vi "Parse Token.vi"(7 "Loader":refnum<class "Abstract.lvclass">, 8 "Error In":errorcluster, 10 "Token":refnum<class "Abstract.lvclass">, 11 "Stack In":refnum<queue>) -> (0 "Error Out":errorcluster, 3 "Stack Out":refnum<queue>)   [LabVIEW 2018, in "Toolkit.lvlib"]
uses:
  Toolkit.lvlib
  Nodes/NonTerminal/NonTerminal.lvclass
  D:/Users/cfield/Code/Field R&D Services/Mustache/LabVIEW/trunk/src/Toolkit/Low-Level/Nodes/Abstract/Abstract.lvclass
  Tokens/Abstract/Abstract.lvclass
  Loaders/Abstract/Abstract.lvclass
  Tokens/Comment/Comment.lvclass
  Tokens/SetDelimiter/SetDelimiter.lvclass
  Tokens/SetDelimiter/SetDelimiter.lvclass/SetDelimiter.ctl
  Tokens/Text/Text.lvclass
  Nodes/Section/Section.lvclass
  D:/Users/cfield/Code/Field R&D Services/Mustache/LabVIEW/trunk/src/Toolkit/Low-Level/Nodes/NonTerminal/NonTerminal.lvclass
  Nodes/Comment/Comment.lvclass
  Nodes/Tag/Tag.lvclass
  Nodes/Partial/Partial.lvclass
  Nodes/Delimiter/Delimiter.lvclass
  Nodes/Text/Text.lvclass
  Lex String.vi
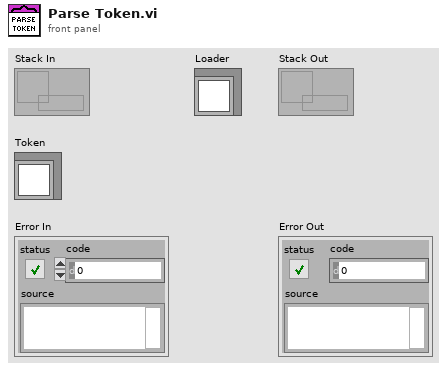
[diagram p1: front panel]
types:
  T1 = typedef "Toolkit.lvlib/Delimiters.ctl" = cluster{"Close":string, "Open":string}
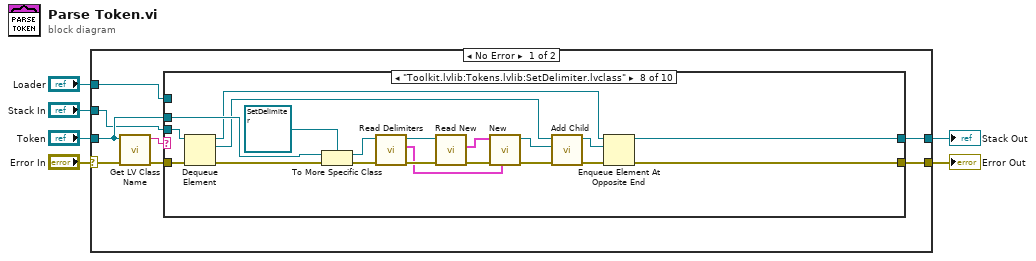
[diagram p0: block diagram]
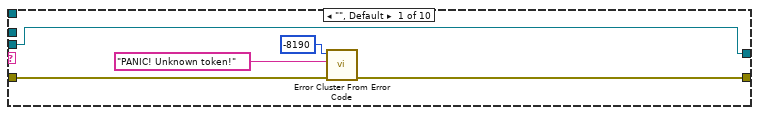
[diagram p2: hidden frame]
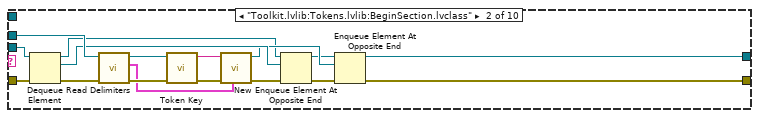
[diagram p3: hidden frame]
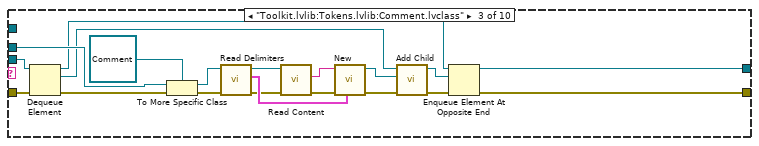
[diagram p4: hidden frame]
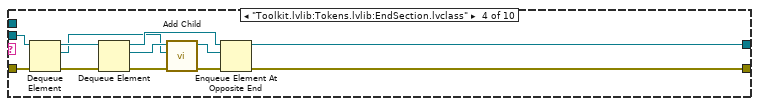
[diagram p5: hidden frame]
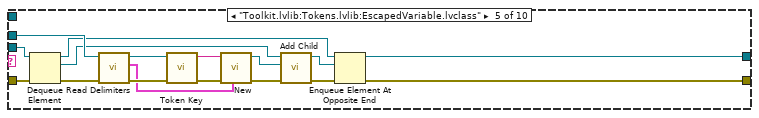
[diagram p6: hidden frame]
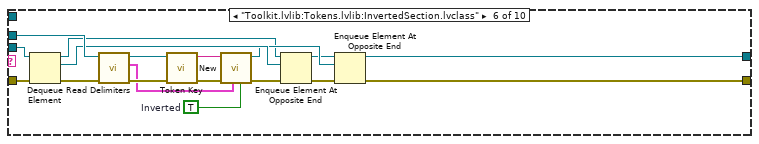
[diagram p7: hidden frame]
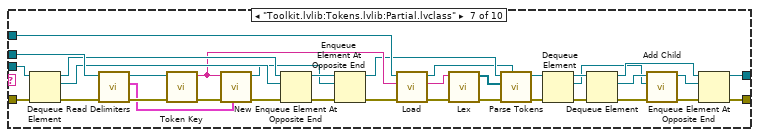
[diagram p8: hidden frame]
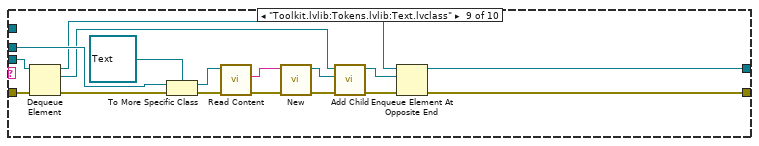
[diagram p9: hidden frame]
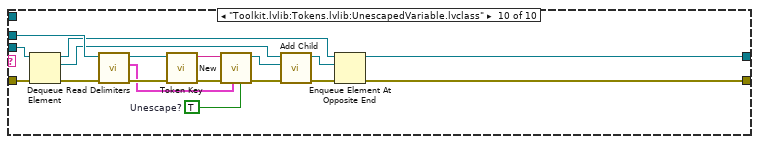
[diagram p10: hidden frame]
diagram:
  n1 = case shown="No Error" "Error In" {
    selector: "Error In" -> [w9 w194]
    tunnel: [w14 w195] -> w6
    tunnel: "Token" -> [w13 _]
    tunnel: [w12 w194] -> w4
    tunnel: "Stack In" -> [w8 w195]
    tunnel: "Loader" -> [w7 _]
    frame No Error {
      n2 = call <vilib>:"Get LV Class Name.vi"("error in (no error)"=w9, "object"=w13) -> ("error out"=w11:errorcluster, "class name"=w10:string)  [unwired: 8 in]
      n3 = case shown="\"Toolkit.lvlib:Tokens.lvlib:SetDelimiter.lvclass\"" w10 {
        tunnel: w11 -> [w19 w33 w56 w68 w85 w100 w136 w158 w175 w191]
        tunnel: [w17 w31 w46 w58 w75 w98 w115 w149 w164 w182] -> w12
        tunnel: w13 -> [_ w36 w55 _ w84 w103 w138 w157 w173 w190]
        tunnel: w8 -> [w15 w34 w52 w67 w81 w101 w137 w155 w170 w188]
        tunnel: [w15 w30 w49 w60 w78 w97 w116 w152 w167 w185] -> w14
        tunnel: w7 -> [_ _ _ _ _ _ w114 _ _ _]
        frame "", Default {
          n4 = call <vilib>:"Error Cluster From Error Code.vi"("error in (no error)"=w19, "error message (\"\")"="PANIC! Unknown token!" ("error message (\"\")"), "error code (0)"=-8190) -> ("error out"=w17:errorcluster)  [unwired: 6 in]
        }
        frame "Toolkit.lvlib:Tokens.lvlib:BeginSection.lvclass" {
          n5 = Dequeue Element(queue=w34, error in (no error)=w33) -> (queue out=w28:refnum<queue>, element=w32:refnum<class "NonTerminal.lvclass">, error out=w22:errorcluster)  [unwired: 1 in, 1 out]
          n6 = call-dynamic "Read Delimiters.vi"("Error In"=w22, "Token In"=w36) -> ("Error Out"=w21:errorcluster, "Delimiters"=w20:T1, "Token Out"=w23:refnum<class "Abstract.lvclass">)  [unwired: 7 in]
          n7 = call "Token Key.vi"("Error In"=w21, "Token"=w23) -> ("Error Out"=w25:errorcluster, "Key"=w35:string)  [unwired: 8 in]
          n8 = call "New.vi"("Delimiters"=w20, "Error In"=w25, "Key"=w35) -> ("Error Out"=w24:errorcluster, "Section"=w29:refnum<class "Section.lvclass">)  [unwired: 7 in]
          n9 = Enqueue Element At Opposite End(queue=w28, element=w32, error in (no error)=w24) -> (queue out=w27:refnum<queue>, error out=w26:errorcluster)  [unwired: 1 in, 1 out]
          n10 = Enqueue Element At Opposite End(queue=w27, element=w29, error in (no error)=w26) -> (queue out=w30:refnum<queue>, error out=w31:errorcluster)  [unwired: 1 in, 1 out]
        }
        frame "Toolkit.lvlib:Tokens.lvlib:Comment.lvclass" {
          n11 = Dequeue Element(queue=w52, error in (no error)=w56) -> (queue out=w50:refnum<queue>, element=w51:refnum<class "NonTerminal.lvclass">, error out=w53:errorcluster)  [unwired: 1 in, 1 out]
          n12 = To More Specific Class(target class=refnum<class "Comment.lvclass"> refnum ("Toolkit.lvlib:Tokens.lvlib:Comment.lvclass"), reference=w55, error in=w53) -> (specific class reference=w41:refnum<class "Comment.lvclass">, error out=w37:errorcluster)
          n13 = call-dynamic "Read Delimiters.vi"("Error In"=w37, "Token In"=w41) -> ("Error Out"=w38:errorcluster, "Delimiters"=w42:T1, "Token Out"=w40:refnum<class "Comment.lvclass">)  [unwired: 7 in]
          n14 = call-dynamic "Read Content.vi"("Error In"=w38, "Contentable In"=w40) -> ("Error Out"=w39:errorcluster, "Content"=w43:string)  [unwired: 7 in, 1 out]
          n15 = call "New.vi"("Delimiters"=w42, "Error In"=w39, "Content"=w43) -> ("Error Out"=w44:errorcluster, "Comment"=w54:refnum<class "Comment.lvclass">)  [unwired: 7 in]
          n16 = call-dynamic "Add Child.vi"("Error In"=w44, "Child"=w54, "Non-Terminal In"=w51) -> ("Error Out"=w47:errorcluster, "Non-Terminal Out"=w48:refnum<class "NonTerminal.lvclass">)  [unwired: 7 in]
          n17 = Enqueue Element At Opposite End(queue=w50, element=w48, error in (no error)=w47) -> (queue out=w49:refnum<queue>, error out=w46:errorcluster)  [unwired: 1 in, 1 out]
        }
        frame "Toolkit.lvlib:Tokens.lvlib:EndSection.lvclass" {
          n18 = Dequeue Element(queue=w67, error in (no error)=w68) -> (queue out=w66:refnum<queue>, element=w62:refnum<class "NonTerminal.lvclass">, error out=w64:errorcluster)  [unwired: 1 in, 1 out]
          n19 = Dequeue Element(queue=w66, error in (no error)=w64) -> (queue out=w65:refnum<queue>, element=w63:refnum<class "NonTerminal.lvclass">, error out=w61:errorcluster)  [unwired: 1 in, 1 out]
          n20 = call-dynamic "Add Child.vi"("Error In"=w61, "Child"=w62, "Non-Terminal In"=w63) -> ("Error Out"=w59:errorcluster, "Non-Terminal Out"=w57:refnum<class "NonTerminal.lvclass">)  [unwired: 7 in]
          n21 = Enqueue Element At Opposite End(queue=w65, element=w57, error in (no error)=w59) -> (queue out=w60:refnum<queue>, error out=w58:errorcluster)  [unwired: 1 in, 1 out]
        }
        frame "Toolkit.lvlib:Tokens.lvlib:EscapedVariable.lvclass" {
          n22 = Dequeue Element(queue=w81, error in (no error)=w85) -> (queue out=w79:refnum<queue>, element=w80:refnum<class "NonTerminal.lvclass">, error out=w71:errorcluster)  [unwired: 1 in, 1 out]
          n23 = call-dynamic "Read Delimiters.vi"("Error In"=w71, "Token In"=w84) -> ("Error Out"=w70:errorcluster, "Delimiters"=w69:T1, "Token Out"=w72:refnum<class "Abstract.lvclass">)  [unwired: 7 in]
          n24 = call "Token Key.vi"("Error In"=w70, "Token"=w72) -> ("Error Out"=w74:errorcluster, "Key"=w82:string)  [unwired: 8 in]
          n25 = call "New.vi"("Delimiters"=w69, "Error In"=w74, "Key"=w82) -> ("Error Out"=w73:errorcluster, "Tag"=w83:refnum<class "Tag.lvclass">)  [unwired: 7 in]
          n26 = call-dynamic "Add Child.vi"("Error In"=w73, "Child"=w83, "Non-Terminal In"=w80) -> ("Error Out"=w76:errorcluster, "Non-Terminal Out"=w77:refnum<class "NonTerminal.lvclass">)  [unwired: 7 in]
          n27 = Enqueue Element At Opposite End(queue=w79, element=w77, error in (no error)=w76) -> (queue out=w78:refnum<queue>, error out=w75:errorcluster)  [unwired: 1 in, 1 out]
        }
        frame "Toolkit.lvlib:Tokens.lvlib:InvertedSection.lvclass" {
          w92 = TRUE  # Inverted
          n28 = Dequeue Element(queue=w101, error in (no error)=w100) -> (queue out=w95:refnum<queue>, element=w99:refnum<class "NonTerminal.lvclass">, error out=w88:errorcluster)  [unwired: 1 in, 1 out]
          n29 = call-dynamic "Read Delimiters.vi"("Error In"=w88, "Token In"=w103) -> ("Error Out"=w87:errorcluster, "Delimiters"=w86:T1, "Token Out"=w89:refnum<class "Abstract.lvclass">)  [unwired: 7 in]
          n30 = call "Token Key.vi"("Error In"=w87, "Token"=w89) -> ("Error Out"=w91:errorcluster, "Key"=w102:string)  [unwired: 8 in]
          n31 = call "New.vi"("Inverted"=w92, "Delimiters"=w86, "Error In"=w91, "Key"=w102) -> ("Error Out"=w90:errorcluster, "Section"=w96:refnum<class "Section.lvclass">)  [unwired: 6 in]
          n32 = Enqueue Element At Opposite End(queue=w95, element=w99, error in (no error)=w90) -> (queue out=w94:refnum<queue>, error out=w93:errorcluster)  [unwired: 1 in, 1 out]
          n33 = Enqueue Element At Opposite End(queue=w94, element=w96, error in (no error)=w93) -> (queue out=w97:refnum<queue>, error out=w98:errorcluster)  [unwired: 1 in, 1 out]
        }
        frame "Toolkit.lvlib:Tokens.lvlib:Partial.lvclass" {
          n34 = Dequeue Element(queue=w137, error in (no error)=w136) -> (queue out=w134:refnum<queue>, element=w135:refnum<class "NonTerminal.lvclass">, error out=w130:errorcluster)  [unwired: 1 in, 1 out]
          n35 = call-dynamic "Read Delimiters.vi"("Error In"=w130, "Token In"=w138) -> ("Error Out"=w129:errorcluster, "Delimiters"=w125:T1, "Token Out"=w131:refnum<class "Abstract.lvclass">)  [unwired: 7 in]
          n36 = call "Token Key.vi"("Error In"=w129, "Token"=w131) -> ("Error Out"=w128:errorcluster, "Key"=w112:string)  [unwired: 8 in]
          n37 = call "New.vi"("Delimiters"=w125, "Error In"=w128, "Key"=w112) -> ("Error Out"=w127:errorcluster, "Partial"=w126:refnum<class "Partial.lvclass">)  [unwired: 7 in]
          n38 = Enqueue Element At Opposite End(queue=w134, element=w135, error in (no error)=w127) -> (queue out=w133:refnum<queue>, error out=w132:errorcluster)  [unwired: 1 in, 1 out]
          n39 = Enqueue Element At Opposite End(queue=w133, element=w126, error in (no error)=w132) -> (queue out=w107:refnum<queue>, error out=w113:errorcluster)  [unwired: 1 in, 1 out]
          n40 = call-dynamic "Load.vi"("Error In"=w113, "Key"=w112, "Loader In"=w114) -> ("Error Out"=w105:errorcluster, "Template"=w106:string, "Loader Out"=w104:refnum<class "Abstract.lvclass">)  [unwired: 6 in]
          n41 = call-poly "Lex.vi"("Error In"=w105, "Input"=w106) -> ("Error Out"=w111:errorcluster, "Tokens"=w110:refnum<class "Abstract.lvclass">[])  [unwired: 8 in]
          n42 = call "Parse Tokens.vi"("Loader"=w104, "Error In"=w111, "Tokens"=w110, "Stack In"=w107) -> ("Error Out"=w109:errorcluster, "Stack Out"=w108:refnum<queue>)  [unwired: 6 in]
          n43 = Dequeue Element(queue=w108, error in (no error)=w109) -> (queue out=w124:refnum<queue>, element=w120:refnum<class "NonTerminal.lvclass">, error out=w122:errorcluster)  [unwired: 1 in, 1 out]
          n44 = Dequeue Element(queue=w124, error in (no error)=w122) -> (queue out=w123:refnum<queue>, element=w121:refnum<class "NonTerminal.lvclass">, error out=w119:errorcluster)  [unwired: 1 in, 1 out]
          n45 = call-dynamic "Add Child.vi"("Error In"=w119, "Child"=w120, "Non-Terminal In"=w121) -> ("Error Out"=w118:errorcluster, "Non-Terminal Out"=w117:refnum<class "NonTerminal.lvclass">)  [unwired: 7 in]
          n46 = Enqueue Element At Opposite End(queue=w123, element=w117, error in (no error)=w118) -> (queue out=w116:refnum<queue>, error out=w115:errorcluster)  [unwired: 1 in, 1 out]
        }
        frame "Toolkit.lvlib:Tokens.lvlib:SetDelimiter.lvclass" {
          n47 = Dequeue Element(queue=w155, error in (no error)=w158) -> (queue out=w153:refnum<queue>, element=w154:refnum<class "NonTerminal.lvclass">, error out=w156:errorcluster)  [unwired: 1 in, 1 out]
          n48 = To More Specific Class(target class=refnum<class "SetDelimiter.lvclass"> refnum ("Toolkit.lvlib:Tokens.lvlib:SetDelimiter.lvclass"), reference=w157, error in=w156) -> (specific class reference=w148:refnum<class "SetDelimiter.lvclass">, error out=w147:errorcluster)
          n49 = call-dynamic "Read Delimiters.vi"("Error In"=w147, "Token In"=w148) -> ("Error Out"=w145:errorcluster, "Delimiters"=w139:T1, "Token Out"=w144:refnum<class "SetDelimiter.lvclass">)  [unwired: 7 in]
          n50 = call "Read New.vi"("Error In"=w145, "SetDelimiter In"=w144) -> ("Error Out"=w143:errorcluster, "New Value"=w140:cluster{"Close":string, "Open":string})  [unwired: 7 in, 1 out]
          n51 = call "New.vi"("Delimiters"=w139, "Error In"=w143, "New Delimiters"=w140) -> ("Error Out"=w142:errorcluster, "Delimiter"=w141:refnum<class "Delimiter.lvclass">)  [unwired: 7 in]
          n52 = call-dynamic "Add Child.vi"("Error In"=w142, "Child"=w141, "Non-Terminal In"=w154) -> ("Error Out"=w150:errorcluster, "Non-Terminal Out"=w151:refnum<class "NonTerminal.lvclass">)  [unwired: 7 in]
          n53 = Enqueue Element At Opposite End(queue=w153, element=w151, error in (no error)=w150) -> (queue out=w152:refnum<queue>, error out=w149:errorcluster)  [unwired: 1 in, 1 out]
        }
        frame "Toolkit.lvlib:Tokens.lvlib:Text.lvclass" {
          n54 = Dequeue Element(queue=w170, error in (no error)=w175) -> (queue out=w168:refnum<queue>, element=w169:refnum<class "NonTerminal.lvclass">, error out=w171:errorcluster)  [unwired: 1 in, 1 out]
          n55 = To More Specific Class(target class=refnum<class "Text.lvclass"> refnum ("Toolkit.lvlib:Tokens.lvlib:Text.lvclass"), reference=w173, error in=w171) -> (specific class reference=w162:refnum<class "Text.lvclass">, error out=w161:errorcluster)
          n56 = call-dynamic "Read Content.vi"("Error In"=w161, "Contentable In"=w162) -> ("Error Out"=w159:errorcluster, "Content"=w160:string)  [unwired: 7 in, 1 out]
          n57 = call "New.vi"("Error In"=w159, "Content"=w160) -> ("Error Out"=w163:errorcluster, "Text"=w172:refnum<class "Text.lvclass">)  [unwired: 8 in]
          n58 = call-dynamic "Add Child.vi"("Error In"=w163, "Child"=w172, "Non-Terminal In"=w169) -> ("Error Out"=w165:errorcluster, "Non-Terminal Out"=w166:refnum<class "NonTerminal.lvclass">)  [unwired: 7 in]
          n59 = Enqueue Element At Opposite End(queue=w168, element=w166, error in (no error)=w165) -> (queue out=w167:refnum<queue>, error out=w164:errorcluster)  [unwired: 1 in, 1 out]
        }
        frame "Toolkit.lvlib:Tokens.lvlib:UnescapedVariable.lvclass" {
          w192 = TRUE  # Unescape?
          n60 = Dequeue Element(queue=w188, error in (no error)=w191) -> (queue out=w186:refnum<queue>, element=w187:refnum<class "NonTerminal.lvclass">, error out=w178:errorcluster)  [unwired: 1 in, 1 out]
          n61 = call-dynamic "Read Delimiters.vi"("Error In"=w178, "Token In"=w190) -> ("Error Out"=w177:errorcluster, "Delimiters"=w176:T1, "Token Out"=w179:refnum<class "Abstract.lvclass">)  [unwired: 7 in]
          n62 = call "Token Key.vi"("Error In"=w177, "Token"=w179) -> ("Error Out"=w181:errorcluster, "Key"=w189:string)  [unwired: 8 in]
          n63 = call "New.vi"("Unescaped"=w192, "Delimiters"=w176, "Error In"=w181, "Key"=w189) -> ("Error Out"=w180:errorcluster, "Tag"=w193:refnum<class "Tag.lvclass">)  [unwired: 6 in]
          n64 = call-dynamic "Add Child.vi"("Error In"=w180, "Child"=w193, "Non-Terminal In"=w187) -> ("Error Out"=w183:errorcluster, "Non-Terminal Out"=w184:refnum<class "NonTerminal.lvclass">)  [unwired: 7 in]
          n65 = Enqueue Element At Opposite End(queue=w186, element=w184, error in (no error)=w183) -> (queue out=w185:refnum<queue>, error out=w182:errorcluster)  [unwired: 1 in, 1 out]
        }
      }
    }
    frame Error {
    }
  }
  "Stack Out" <- w6
  "Error Out" <- w4
